vi "Update Thing Shadow.vi"(6 "Version":i32, 8 "error in (no error)":errorcluster, 9 "Reported State":T1[](array[typedef]), 10 "Desired State":T1[](array[typedef]), 11 "Thing Shadow in":refnum<class "Thing Shadow.lvclass">) -> (0 "error out":errorcluster, 3 "Thing Shadow out":refnum<class "Thing Shadow.lvclass">)   [LabVIEW 2015, in "NI_AWS_IoT.lvlib" / "Thing Shadow.lvclass"]
uses:
  Thing Shadow.lvclass
  JSON Parsing/Name-Value with Type.ctl
  JSON Parsing/Name Value Pair.ctl
  JSON Parsing/JSON Type.ctl
  Core/HTTP Request/Request Options.ctl
  Core/HTTP Request/Name Value Pair.ctl
  Core/HTTP Request/Region handling.ctl
  Core/HTTP Request/URL formatting.ctl
  Thing Shadow.lvclass/Thing Shadow.ctl
  Read Thing Name.vi
  Core/HTTP Request/HTTP Request.lvclass
  NI_AWS_IoT.lvlib
  JSON Parsing/NI_JSON Parsing.lvlib
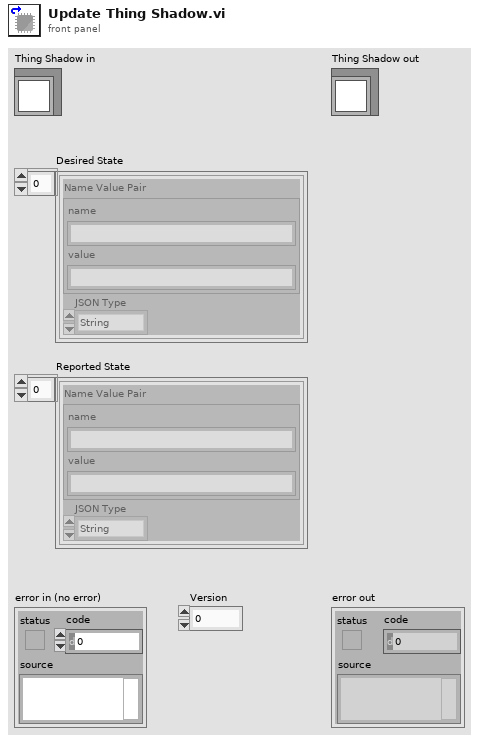
[diagram p1: front panel]
types:
  T1 = typedef "NI_JSON Parsing.lvlib/Name-Value with Type.ctl" = cluster{"Name Value Pair":T2, "JSON Type":T3}
  T2 = typedef "NI_JSON Parsing.lvlib/Name Value Pair.ctl" = cluster{"name":string, "value":string}
  T3 = typedef "NI_JSON Parsing.lvlib/JSON Type.ctl" = enum16{"String", "Numeric", "Boolean"}
  T4 = typedef "NI_AWS_Core.lvlib/HTTP Request.lvclass/Name Value Pair.ctl" = cluster{"name":string, "value":string}
  T5 = typedef "NI_AWS_Core.lvlib/HTTP Request.lvclass/Request Options.ctl" = cluster{"request headers":T4[], "request parameters":T4[], "request body":string, "region handling":T6, "URL formatting":T7}
  T6 = typedef "NI_AWS_Core.lvlib/HTTP Request.lvclass/Region handling.ctl" = enum16{"use region everywhere", "use region (authentication only)", "use region (URL only)", "ignore region everwhere"}
  T7 = typedef "NI_AWS_Core.lvlib/HTTP Request.lvclass/URL formatting.ctl" = enum16{"region-", "region."}
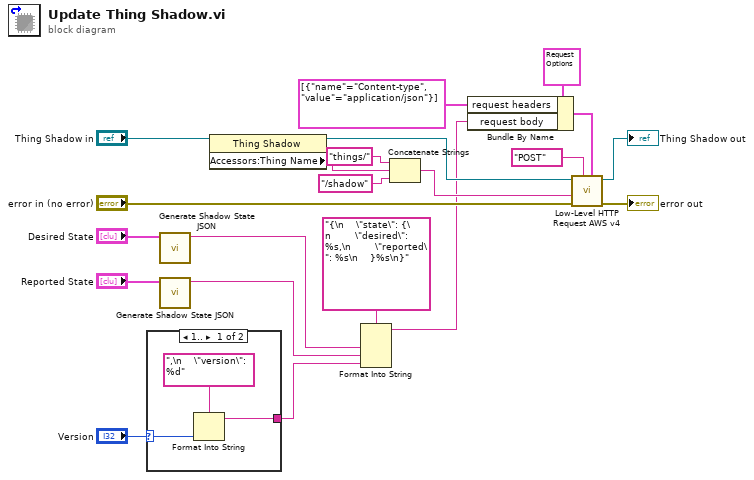
[diagram p0: block diagram]
diagram:
  n1 = case shown="1.." "Version" {
    selector: "Version" -> [w23 _]
    tunnel: [w22 _] -> w1
    frame 1.. {
      n2 = Format Into String(format string=",\n    \"version\": %d", w23) -> (resulting string=w22:string)  [unwired: 2 in, 1 out]
    }
    frame ..0 {
    }
  }
  n3 = call "Generate Shadow State JSON.vi"("State"="Desired State") -> ("JSON"=w3:string)  [unwired: 10 in]
  n4 = call "Generate Shadow State JSON.vi"("State"="Reported State") -> ("JSON"=w4:string)  [unwired: 10 in]
  n5 = property class="Thing Shadow"(reference="Thing Shadow in") -> (reference out=w11:refnum<class "Thing Shadow.lvclass">, "Accessors:Thing Name"=w2:string)  [unwired: 1 in, 1 out]
  n6 = Format Into String(format string="{\n    \"state\": {\n        \"desired\": %s,\n        \"reported\": %s\n    }%s\n}", w3, w4, w1) -> (resulting string=w8:string)  [unwired: 2 in, 1 out]
  n7 = Concatenate Strings("things/" ("string"), w2, "/shadow" ("string")) -> (w15:string)
  n8 = Bundle By Name(cluster=T5 {"request headers"=[], "request parameters"=[], "request body"="", "region handling"=enum."use region everywhere", "URL formatting"=enum."region."} ("Request Options"), "request headers"=T4[] [{"name"="Content-type", "value"="application/json"}], "request body"=w8) -> (w16:T5)
  n9 = call "Low-Level HTTP Request AWS v4.vi"("Request Options"=w16, "HTTP-Verb"="POST", "error in (no error)"="error in (no error)", "URL Suffix"=w15, "AWS Core in"=w11) -> ("error out"=→"error out":errorcluster, "AWS Core out"=→"Thing Shadow out":refnum<class "Thing Shadow.lvclass">)  [unwired: 3 in, 2 out]
